vi "MergeColorPlanes.vi"(9 "Blue":T1, 10 "Green":T1, 11 "Red":T1) -> (3 "image data":T1)   [LabVIEW 2019]
uses:
  <vilib>/picture/picture.llb/imagedata.ctl
panel:
  out "image size":i32
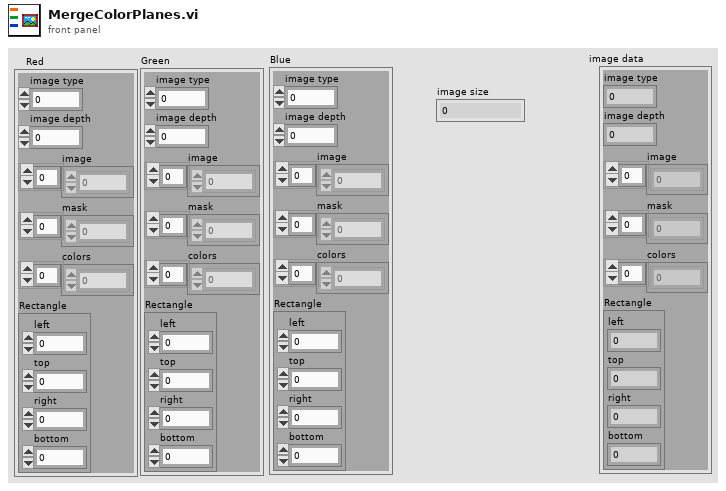
[diagram p1: front panel]
types:
  T1 = typedef "imagedata.ctl" = cluster{"image type":i32, "image depth":i32, "image":u8[], "mask":u8[], "colors":u32[], "Rectangle":cluster{"left":i16, "top":i16, "right":i16, "bottom":i16}}
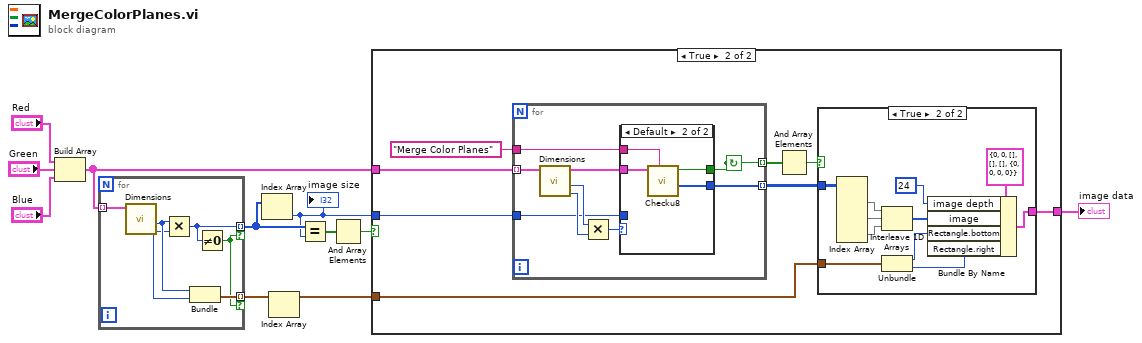
[diagram p0: block diagram]
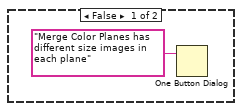
[diagram p2: hidden frame]
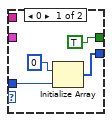
[diagram p3: hidden frame]
diagram:
  n1 = Build Array("Red", "Green", "Blue") -> (w5:T1[])
  n2 = for {
    tunnel: w5 -> [w17] mode=indexing
    tunnel: [w16] -> w8 mode=indexing if=w12
    tunnel: [w13] -> w1 mode=indexing if=w12
    n3 = call "Dimensions.vi"("Image In"=w17) -> ("width"=w14:i32, "height"=w15:i32)  [unwired: 8 in, 1 out]
    n4 = Multiply(x=w15, y=w14) -> (x*y=w16:i32)
    n5 = Bundle("height"=w15, "width"=w14) -> (w13:cluster{"height":i32, "width":i32})  [unwired: 1 in]
    n6 = Not Equal To 0?(x=w16) -> (x != 0?=w12:bool)
  }
  n7 = Index Array(array=w8) -> (element=w3:i32)  [unwired: 1 in]
  "image size" <- w3
  n8 = Index Array(array=w1) -> (element=w2:cluster{"height":i32, "width":i32})  [unwired: 1 in]
  n9 = Equal?(x=w8, y=w3) -> (x = y?=w7:bool[])
  n10 = And Array Elements(Boolean array=w7) -> (logical AND=w6:bool)
  n11 = case shown="True" w6 {
    tunnel: w5 -> [_ w22]
    tunnel: [_ w21] -> w4
    tunnel: w3 -> [_ w20]
    tunnel: w2 -> [_ w19]
    frame False {
      n12 = One Button Dialog(message="Merge Color Planes has different size images in each plane") -> ()  [unwired: 1 in, 1 out]
    }
    frame True {
      n13 = for {
        tunnel: "Merge Color Planes" ("input 1") -> [w35]
        tunnel: [w28] -> w25 mode=indexing
        tunnel: [w34] -> w24 mode=indexing
        tunnel: w22 -> [w29] mode=indexing
        tunnel: w20 -> [w27]
        stop <- w28 continue-if-true
        n14 = call "Dimensions.vi"("Image In"=w29) -> ("width"=w31:i32, "height"=w32:i32, "Image out"=w33:T1)  [unwired: 8 in]
        n15 = Multiply(x=w32, y=w31) -> (x*y=w30:i32)
        n16 = case shown="Default" w30 {
          tunnel: w35 -> [_ w43]
          tunnel: [TRUE ("Success") w42] -> w28
          tunnel: [w38 w41] -> w34
          tunnel: w33 -> [_ w40]
          tunnel: w27 -> [w36 _]
          frame 0 {
            n17 = Initialize Array(u8 0 ("image depth"), w36) -> (w38:u8[])
          }
          frame Default {
            n18 = call "Checku8.vi"("Name"=w43, "Red"=w40) -> ("image"=w41:u8[], "Success"=w42:bool)  [unwired: 8 in]
          }
        }
      }
      n19 = And Array Elements(Boolean array=w25) -> (logical AND=w26:bool)
      n20 = case shown="True" w26 {
        tunnel: w24 -> [_ w50]
        tunnel: [_ w52] -> w21
        tunnel: w19 -> [_ w46]
        frame False {
        }
        frame True {
          n21 = Index Array(array=w50) -> (element #1=w47:u8[], element #2=w48:u8[], element #3=w49:u8[])  [unwired: 6 in]
          n22 = Interleave 1D Arrays(w47, w48, w49) -> (w54:u8[])
          n23 = Unbundle(w46) -> ("height"=w45:i32, "width"=w44:i32)
          n24 = Bundle By Name(cluster=T1 {"image type"=0, "image depth"=0, "image"=[], "mask"=[], "colors"=[], "Rectangle"={"left"=0, "top"=0, "right"=0, "bottom"=0}} ("Red"), "image depth"=24, "image"=w54, "Rectangle.bottom"=w45, "Rectangle.right"=w44) -> (w52:T1)
        }
      }
    }
  }
  "image data" <- w4
